vi "Render.vi"(8 "error in":errorcluster, 10 "Renderer in":refnum<class "Renderer.lvclass">, 11 "Dqmh Modules Overview":refnum<class "Dqmh Modules Overview.lvclass">) -> (0 "error out":errorcluster, 3 "Sections out":refnum<class "Section.lvclass">[](array[class]))   [LabVIEW 2021, in "TAF Proj Document Type.lvlib" / "Dqmh Modules Overview.lvclass"]
uses:
  <vilib>/Wovalab/AntiDoc/Document Type/Add-ons/LabVIEW TAF Project/Dqmh Modules Overview/Dqmh Modules Overview.lvclass
  C:/Program Files (x86)/National Instruments/LabVIEW 2021/vi.lib/Wovalab/AntiDoc/Bloc/Bloc.lvclass
  <vilib>/Wovalab/AsciiDoc for LabVIEW/Section/Section.lvclass
  <vilib>/Wovalab/AntiDoc/Renderer/Renderer.lvclass
  <vilib>/Wovalab/AsciiDoc for LabVIEW/Diagram/Type--enum.ctl
  <vilib>/Wovalab/AntiDoc/GraphBuilder/Graph/Graph.lvclass
  <vilib>/Wovalab/AntiDoc/GraphBuilder/Renderer/Graphviz/Graphviz.lvclass
  C:/Program Files (x86)/National Instruments/LabVIEW 2021/vi.lib/Wovalab/AntiDoc/GraphBuilder/Renderer/Renderer.lvclass
  <vilib>/Wovalab/AntiDoc/GraphBuilder/Shapes/Edge/Graphviz/Graphviz Edge Shape.lvclass
  <vilib>/Wovalab/AntiDoc/GraphBuilder/Shapes/Node/Graphviz/Graphviz Node Shape.lvclass
  <vilib>/Wovalab/AntiDoc/GraphBuilder/Shapes/Edge/Graphviz/Shape.ctl
  <vilib>/Wovalab/AntiDoc/GraphBuilder/Shapes/Edge/Graphviz/Colors.ctl
  <vilib>/Wovalab/AntiDoc/GraphBuilder/Shapes/Node/Graphviz/Colors.ctl
  <vilib>/Wovalab/AntiDoc/GraphBuilder/Shapes/Node/Graphviz/Shape.ctl
  <vilib>/Wovalab/AntiDoc/GraphBuilder/Renderer/Graphviz/Graph Direction.ctl
  <vilib>/Wovalab/AntiDoc/Document Type/Add-ons/LabVIEW TAF Project/Dqmh Modules Overview/Dqmh Modules Overview.lvclass/Dqmh Modules Overview.ctl
  <vilib>/Wovalab/AntiDoc/Bloc/Bloc.lvclass/Bloc.ctl
  <vilib>/Wovalab/AntiDoc/Document Type/Add-ons/LabVIEW TAF Project/Dqmh Modules Overview/Link Type--enum.ctl
  <vilib>/Wovalab/AntiDoc/Document Type/Add-ons/LabVIEW TAF Project/Dqmh Module/Dqmh Module.lvclass/Dqmh Module.ctl
  <vilib>/Wovalab/AsciiDoc for LabVIEW/Table/Table.lvclass/Table.ctl
  <vilib>/Wovalab/AntiDoc/Document Type/Add-ons/LabVIEW TAF Project/Dqmh Module/Read Dqmh Module Type.vi
  <vilib>/Wovalab/AntiDoc/Bloc/Read Name.vi
  <vilib>/Wovalab/AntiDoc/Document Type/Add-ons/LabVIEW TAF Project/Dqmh Module/Read Start Module Callers.vi
  <vilib>/Wovalab/AntiDoc/Document Type/Add-ons/LabVIEW TAF Project/Dqmh Module/Read Stop Module Callers.vi
  <vilib>/Wovalab/AntiDoc/Document Type/Add-ons/LabVIEW TAF Project/Dqmh Module/Read Request Link.vi
  <vilib>/Wovalab/AntiDoc/Document Type/Add-ons/LabVIEW TAF Project/Dqmh Module/Read Request With Reply Links.vi
  <vilib>/Wovalab/AntiDoc/Document Type/Add-ons/LabVIEW TAF Project/Dqmh Module/Read Broadcast Link.vi
  <vilib>/Wovalab/AntiDoc/Document Type/Add-ons/LabVIEW TAF Project/Dqmh Module/Dqmh Module.lvclass
  <vilib>/Wovalab/AsciiDoc for LabVIEW/Paragraph/Paragraph.lvclass
  C:/Program Files (x86)/National Instruments/LabVIEW 2021/vi.lib/Wovalab/AsciiDoc for LabVIEW/Adoc-Bloc/Bloc.lvclass
  <vilib>/Wovalab/AsciiDoc for LabVIEW/Table/Table.lvclass
  <vilib>/Wovalab/AsciiDoc for LabVIEW/Diagram/Diagram.lvclass
  <vilib>/Wovalab/AsciiDoc for LabVIEW/Section/Add Bloc (array).vi
  <vilib>/Wovalab/AntiDoc/Document Type/Add-ons/LabVIEW TAF Project/TAF Proj Document Type.lvlib
  <vilib>/Wovalab/AntiDoc/Utilities/Utilities.lvlib
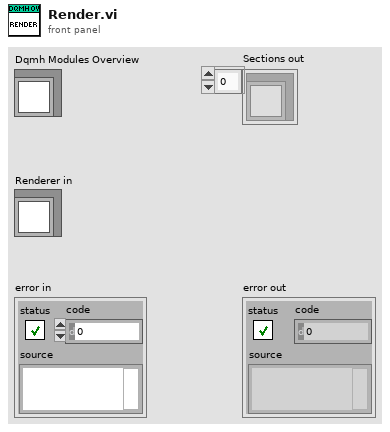
[diagram p1: front panel]
types:
  T1 = typedef "GraphBuilder.lvlib/Graphviz.lvclass/Graph Direction.ctl" = enum16{"Top to Bottom", "Left To Right", "Bottom to Top", "Right to Left"}
  T2 = typedef "GraphBuilder.lvlib/Graphviz Node Shape.lvclass/Shape.ctl" = enum16{"box", "polygon", "ellipse", "oval", "circle", "point", "egg", "triangle", "plaintext", "plain", "diamond", "trapezium", "parallelogram", "house", "pentagon", "hexagon", "septagon", "octagon", "doublecircle", "doubleoctagon", "tripleoctagon", "invtriangle", "invtrapezium", "invhouse", "Mdiamond", "Msquare", "Mcircle", "rect", "rectangle", "square", "star", "none", "underline", "cylinder", "note", "tab", "folder", "box3D", "component", "promoter", "cds", "terminator", "utr", "primersite", "restrictionsite", "fivepoverhang", "threepoverhang", "noverhang", "assembly", "signature", "insulator", "ribosite", "rnastab", "proteasesite", "proteinstab", "rpromoter", "rarrow", "larrow", "lpromoter"}
  T3 = typedef "GraphBuilder.lvlib/Graphviz Node Shape.lvclass/Colors.ctl" = enum16{"aliceblue", "antiquewhite", "aqua", "aquamarine", "azure", "beige", "bisque", "black", "blanchedalmond", "blue", "blueviolet", "brown", "burlywood", "cadetblue", "chartreuse", "chocolate", "coral", "cornflowerblue", "cornsilk", "crimson", "cyan", "darkblue", "darkcyan", "darkgoldenrod", "darkgray", "darkgreen", "darkgrey", "darkkhaki", "darkmagenta", "darkolivegreen", "darkorange", "darkorchid", "darkred", "darksalmon", "darkseagreen", "darkslateblue", "darkslategray", "darkslategrey", "darkturquoise", "darkviolet", "deeppink", "deepskyblue", "dimgray", "dimgrey", "dodgerblue", "firebrick", "floralwhite", "forestgreen", "fuchsia", "gainsboro", "ghostwhite", "gold", "goldenrod", "gray", "green", "greenyellow", "grey", "honeydew", "hotpink", "indianred", "indigo", "ivory", "khaki", "lavender", "lavenderblush", "lawngreen", "lemonchiffon", "lightblue", "lightcoral", "lightcyan", "lightgoldenrodyellow", "lightgray", "lightgreen", "lightgrey", "lightpink", "lightsalmon", "lightseagreen", "lightskyblue", "lightslategray", "lightslategrey", "lightsteelblue", "lightyellow", "lime", "limegreen", "linen", "magenta", "maroon", "mediumaquamarine", "mediumblue", "mediumorchid", "mediumpurple", "mediumseagreen", "mediumslateblue", "mediumspringgreen", "mediumturquoise", "mediumvioletred", "midnightblue", "mintcream", "mistyrose", "moccasin", "navajowhite", "navy", "oldlace", "olive", "olivedrab", "orange", "orangered", "orchid", "palegoldenrod", "palegreen", "paleturquoise", "palevioletred", "papayawhip", "peachpuff", "peru", "pink", "plum", "powderblue", "purple", "red", "rosybrown", "royalblue", "saddlebrown", "salmon", "sandybrown", "seagreen", "seashell", "sienna", "silver", "skyblue", "slateblue", "slategray", "slategrey", "snow", "springgreen", "steelblue", "tan", "teal", "thistle", "tomato", "turquoise", "violet", "wheat", "white", "whitesmoke", "yellow", "yellowgreen"}
  T4 = typedef "GraphBuilder.lvlib/Graphviz Edge Shape.lvclass/Colors.ctl" = enum16{"aliceblue", "antiquewhite", "aqua", "aquamarine", "azure", "beige", "bisque", "black", "blanchedalmond", "blue", "blueviolet", "brown", "burlywood", "cadetblue", "chartreuse", "chocolate", "coral", "cornflowerblue", "cornsilk", "crimson", "cyan", "darkblue", "darkcyan", "darkgoldenrod", "darkgray", "darkgreen", "darkgrey", "darkkhaki", "darkmagenta", "darkolivegreen", "darkorange", "darkorchid", "darkred", "darksalmon", "darkseagreen", "darkslateblue", "darkslategray", "darkslategrey", "darkturquoise", "darkviolet", "deeppink", "deepskyblue", "dimgray", "dimgrey", "dodgerblue", "firebrick", "floralwhite", "forestgreen", "fuchsia", "gainsboro", "ghostwhite", "gold", "goldenrod", "gray", "green", "greenyellow", "grey", "honeydew", "hotpink", "indianred", "indigo", "ivory", "khaki", "lavender", "lavenderblush", "lawngreen", "lemonchiffon", "lightblue", "lightcoral", "lightcyan", "lightgoldenrodyellow", "lightgray", "lightgreen", "lightgrey", "lightpink", "lightsalmon", "lightseagreen", "lightskyblue", "lightslategray", "lightslategrey", "lightsteelblue", "lightyellow", "lime", "limegreen", "linen", "magenta", "maroon", "mediumaquamarine", "mediumblue", "mediumorchid", "mediumpurple", "mediumseagreen", "mediumslateblue", "mediumspringgreen", "mediumturquoise", "mediumvioletred", "midnightblue", "mintcream", "mistyrose", "moccasin", "navajowhite", "navy", "oldlace", "olive", "olivedrab", "orange", "orangered", "orchid", "palegoldenrod", "palegreen", "paleturquoise", "palevioletred", "papayawhip", "peachpuff", "peru", "pink", "plum", "powderblue", "purple", "red", "rosybrown", "royalblue", "saddlebrown", "salmon", "sandybrown", "seagreen", "seashell", "sienna", "silver", "skyblue", "slateblue", "slategray", "slategrey", "snow", "springgreen", "steelblue", "tan", "teal", "thistle", "tomato", "turquoise", "violet", "wheat", "white", "whitesmoke", "yellow", "yellowgreen"}
  T5 = typedef "GraphBuilder.lvlib/Graphviz Edge Shape.lvclass/Shape.ctl" = enum16{"box", "lbox", "rbox", "obox", "olbox", "orbox", "crow", "lcrow", "rcrow", "diamond", "ldiamond", "rdiamond", "odiamond", "oldiamond", "ordiamond", "dot", "odot", "inv", "linv", "rinv", "oinv", "olinv", "orinv", "none", "normal", "lnormal", "rnormal", "onormal", "olnormal", "ornormal", "tee", "ltee", "rtee", "vee", "lvee", "rvee", "curve", "lcurve", "rcurve", "icurve", "licurve", "ricurve"}
  T6 = typedef "Wovalab_lib_AsciiDoctor.lvlib/Diagram.lvclass/Type--enum.ctl" = enum16{"a2s", "actdiag", "blockdiag", "ditaa", "erd", "graphviz", "meme", "mermaid", "msc", "nwdiag", "packetdiag", "plantuml", "rackdiag", "seqdiag", "shaape", "svgbob", "syntrax", "umlet", "vega", "vegalite", "wavedrom"}
  T7 = typedef "TAF Proj Document Type.lvlib/Dqmh Modules Overview.lvclass/Link Type--enum.ctl" = enum16{"Request", "Broadcast", "Request With Reply"}
  T8 = typedef "TAF Proj Document Type.lvlib/Project Parser.lvlib/Dqmh Module Type--enum.ctl" = enum16{"Singleton", "Cloneable"}
  T9 = typedef "TAF Proj Document Type.lvlib/Dqmh Module.lvclass/Event Callers--cluster.ctl" = cluster{"Event Name":string, "Caller Names":string[]}
  T10 = typedef "GraphBuilder.lvlib/Graphviz.lvclass/Specific Edge Shape Def.ctl" = cluster{"Source Node ID":string, "Target Node ID":string, "Caption":string, "Graphviz Edge Shape":refnum<class "Graphviz Edge Shape.lvclass">}
  T11 = typedef "GraphBuilder.lvlib/Graphviz.lvclass/Specific Node Shape Def.ctl" = cluster{"Node ID":string, "Graphviz Node Shape":refnum<class "Graphviz Node Shape.lvclass">}
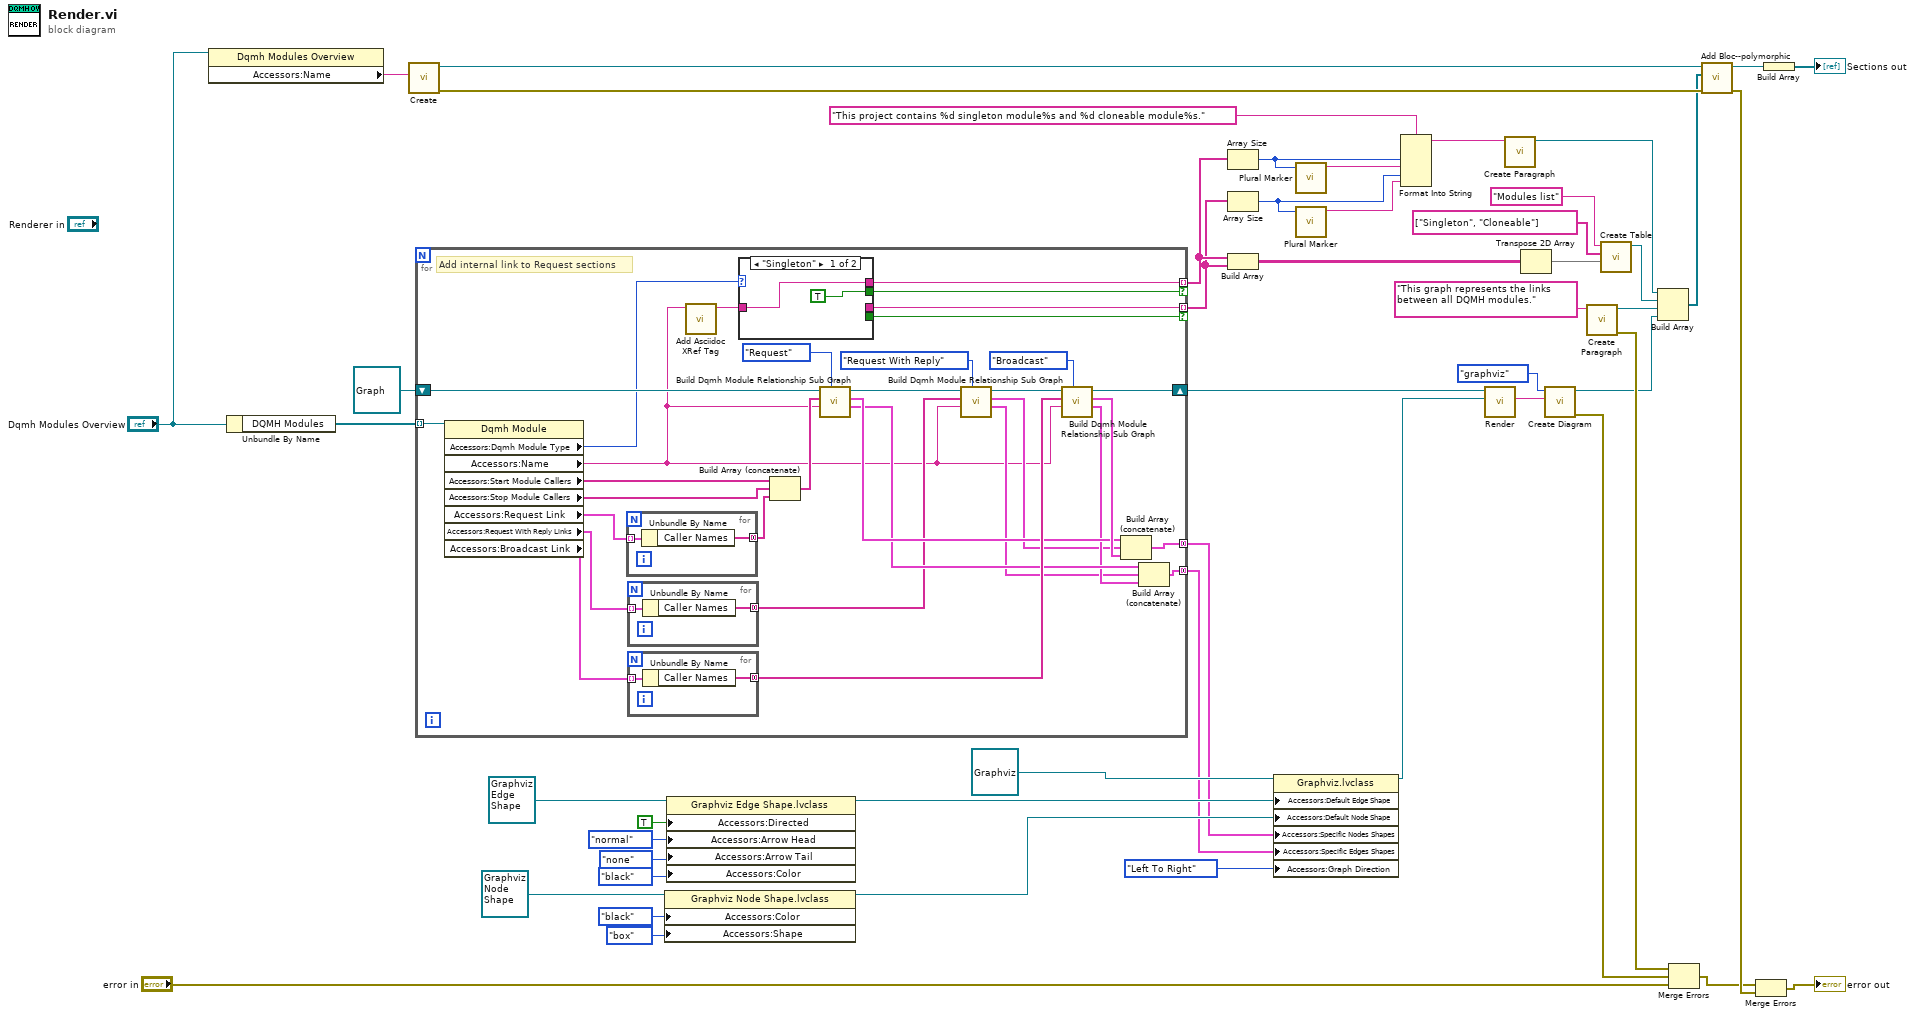
[diagram p0: block diagram]
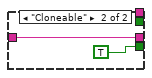
[diagram p2: hidden frame]
diagram:
  n1 = property class="Dqmh Modules Overview"(reference="Dqmh Modules Overview") -> ("Accessors:Name"=w3:string)  [unwired: 1 in, 2 out]
  n2 = Unbundle By Name("Dqmh Modules Overview") -> ("DQMH Modules"=w39:refnum<class "Dqmh Module.lvclass">[])
  n3 = call <vilib>:"Create.vi"("Title"=w3) -> ("error out"=w46:errorcluster, "Section out"=w43:refnum<class "Section.lvclass">)  [unwired: 9 in]
  n4 = for {
    tunnel: w39 -> [w82] mode=indexing
    shift-right: [w74] -> w23
    shift-left: refnum<class "Graph.lvclass"> refnum ("GraphBuilder.lvlib:Graph.lvclass") -> [w75]
    tunnel: [w67] -> w26 mode=concatenating
    tunnel: [w66] -> w25 mode=concatenating
    tunnel: [w64] -> w9 mode=indexing if=w62
    tunnel: [w63] -> w10 mode=indexing if=w61
    # "Add internal link to Request sections"
    n5 = property class="Dqmh Module"(reference=w82) -> ("Accessors:Dqmh Module Type"=w65:T8, "Accessors:Name"=w52:string, "Accessors:Start Module Callers"=w81:string[], "Accessors:Stop Module Callers"=w80:string[], "Accessors:Request Link"=w60:T9[], "Accessors:Request With Reply Links"=w56:T9[], "Accessors:Broadcast Link"=w78:T9[])  [unwired: 1 in, 2 out]
    n6 = for {
      tunnel: w60 -> [w92] mode=indexing
      tunnel: [w91] -> w79 mode=concatenating
      n7 = Unbundle By Name(w92) -> ("Caller Names"=w91:string[])
    }
    n8 = for {
      tunnel: w56 -> [w84] mode=indexing
      tunnel: [w83] -> w55 mode=concatenating
      n9 = Unbundle By Name(w84) -> ("Caller Names"=w83:string[])
    }
    n10 = for {
      tunnel: w78 -> [w90] mode=indexing
      tunnel: [w89] -> w72 mode=concatenating
      n11 = Unbundle By Name(w90) -> ("Caller Names"=w89:string[])
    }
    n12 = call <vilib>:"Add Asciidoc XRef Tag.vi"("String In"=w52) -> ("String out"=w51:string)  [unwired: 10 in]
    n13 = case shown="\"Singleton\"" w65 {
      tunnel: [_ w88] -> w64
      tunnel: w51 -> [w86 w88]
      tunnel: [w86 _] -> w63
      tunnel: [_ TRUE] -> w62
      tunnel: [TRUE _] -> w61
      frame "Singleton" {
      }
      frame "Cloneable" {
      }
    }
    n14 = Build Array (concatenate)(w81, w80, w79) -> (w77:string[])
    n15 = call <vilib>:"Build Dqmh Module Relationship Sub Graph.vi"("Link Type"=Link_Type--enum."Request", "Module Name"=w52, "Caller Names"=w77, "Graph in"=w75) -> ("Specific Edge Shape"=w69:T10[], "Specific Node Shape"=w70:T11[], "Graph out"=w59:refnum<class "Graph.lvclass">)  [unwired: 5 in]
    n16 = call <vilib>:"Build Dqmh Module Relationship Sub Graph.vi"("Link Type"=Link_Type--enum."Request With Reply", "Module Name"=w52, "Caller Names"=w55, "Graph in"=w59) -> ("Specific Edge Shape"=w53:T10[], "Specific Node Shape"=w54:T11[], "Graph out"=w58:refnum<class "Graph.lvclass">)  [unwired: 5 in]
    n17 = call <vilib>:"Build Dqmh Module Relationship Sub Graph.vi"("Link Type"=Link_Type--enum."Broadcast", "Module Name"=w52, "Caller Names"=w72, "Graph in"=w58) -> ("Specific Edge Shape"=w68:T10[], "Specific Node Shape"=w71:T11[], "Graph out"=w74:refnum<class "Graph.lvclass">)  [unwired: 5 in]
    n18 = Build Array (concatenate)(w70, w54, w71) -> (w67:T11[])
    n19 = Build Array (concatenate)(w69, w53, w68) -> (w66:T10[])
  }
  n20 = property class="Graphviz Node Shape.lvclass"(reference=refnum<class "Graphviz Node Shape.lvclass"> refnum ("GraphBuilder.lvlib:Graphviz Node Shape.lvclass"), "Accessors:Color"=Colors."black" ("Color"), "Accessors:Shape"=Shape."box" ("Shape")) -> (reference out=w37:refnum<class "Graphviz Node Shape.lvclass">)  [unwired: 1 in, 1 out]
  n21 = property class="Graphviz Edge Shape.lvclass"(reference=refnum<class "Graphviz Edge Shape.lvclass"> refnum ("GraphBuilder.lvlib:Graphviz Edge Shape.lvclass"), "Accessors:Directed"=TRUE ("Directed"), "Accessors:Arrow Head"=Shape."normal" ("Arrow Head"), "Accessors:Arrow Tail"=Shape."none" ("Arrow Tail"), "Accessors:Color"=Colors."black" ("Color")) -> (reference out=w36:refnum<class "Graphviz Edge Shape.lvclass">)  [unwired: 1 in, 1 out]
  n22 = Array Size(array=w10) -> (size(s)=w7:i32)
  n23 = Array Size(array=w9) -> (size(s)=w6:i32)
  n24 = Build Array(w10, w9) -> (w16:string[][])
  n25 = property class="Graphviz.lvclass"(reference=refnum<class "Graphviz.lvclass"> refnum ("GraphBuilder.lvlib:Graphviz.lvclass"), "Accessors:Default Edge Shape"=w36, "Accessors:Default Node Shape"=w37, "Accessors:Specific Nodes Shapes"=w26, "Accessors:Specific Edges Shapes"=w25, "Accessors:Graph Direction"=Graph_Direction."Left To Right" ("Graph Direction")) -> (reference out=w24:refnum<class "Graphviz.lvclass">)  [unwired: 1 in, 1 out]
  n26 = call <vilib>:"Plural Marker.vi"("Size"=w7) -> ("Plural Mark"=w8:string)  [unwired: 10 in]
  n27 = call <vilib>:"Plural Marker.vi"("Size"=w6) -> ("Plural Mark"=w5:string)  [unwired: 10 in]
  n28 = Format Into String(format string="This project contains %d singleton module%s and %d cloneable module%s." ("Content"), w7, w8, w6, w5) -> (resulting string=w11:string)  [unwired: 2 in, 1 out]
  n29 = call-dynamic "Render.vi"("Renderer"=w24, "Graph in"=w23) -> ("Rendered Stream"=w22:string)  [unwired: 7 in, 2 out]
  n30 = call <vilib>:"Create Paragraph.vi"("Content"=w11) -> ("Paragraph out"=w13:refnum<class "Paragraph.lvclass">)  [unwired: 9 in, 1 out]
  n31 = Transpose 2D Array(2D array=w16) -> (transposed array=w15:string[][])
  n32 = call <vilib>:"Create Diagram.vi"("Diagram Source Code"=w22, "Diagram Type"=Type--enum."graphviz") -> ("error out"=w44:errorcluster, "Diagram out"=w20:refnum<class "Diagram.lvclass">)  [unwired: 8 in]
  n33 = call <vilib>:"Create Paragraph.vi"("Content"="This graph represents the links between all DQMH modules.") -> ("error out"=w45:errorcluster, "Paragraph out"=w41:refnum<class "Paragraph.lvclass">)  [unwired: 9 in]
  n34 = call <vilib>:"Create Table.vi"("Content"=w15, "Header"=string[] ["Singleton", "Cloneable"], "Title"="Modules list") -> ("Table out"=w17:refnum<class "Table.lvclass">)  [unwired: 7 in, 1 out]
  n35 = Build Array(w13, w17, w41, w20) -> (w42:refnum<class "Bloc.lvclass">[])
  n36 = Merge Errors(w45, w44, "error in") -> (w48:errorcluster)
  n37 = call-poly <vilib>:"Add Bloc--polymorphic.vi"("error in"=w46, "Bloc"=w42, "Section in"=w43) -> ("error out"=w50:errorcluster, "Section out"=w2:refnum<class "Section.lvclass">)  [unwired: 7 in]
  n38 = Merge Errors(w48, w50) -> (→"error out":errorcluster)
  n39 = Build Array(w2) -> (→"Sections out":refnum<class "Section.lvclass">[])
